vi "Controller - Child 1 -  GET.vi"(8 "error in":errorcluster) -> (0 "error out":errorcluster, 2 "value":dbl)   [LabVIEW 2023, in "Controller.lvlib" / "Controller.lvclass"]
uses:
  Controller.lvclass
  Controller - Ctrl - Actor - Selector.ctl
  GUI/Usr Ev/GUI - Ctrl - Enum - Events.ctl
  GUI/GUI_Class.lvclass
panel:
  in  "Actor Selector":T1=enum."GUI"
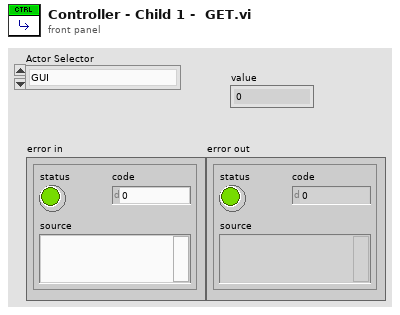
[diagram p1: front panel]
types:
  T1 = typedef "Controller.lvlib/Controller.lvclass/Controller - Ctrl - Actor - Selector.ctl" = enum16{"DISTRIBUTOR", "GUI", "CONSOLE", "SW_INTERFACE", "LOGGING", "ERROR_ENGINE", "EMBEDDED_DB"}
  T2 = typedef "GUI_Actor.lvlib/GUI_Class.lvclass/GUI - Ctrl - Enum - Events.ctl" = enum16{"SEND MESSAGE Ev", "STOP_ACTOR Ev", "INIT_ACTOR Ev", "START Ev", "STOP Ev", "GET Ev", "SET Ev", "ERROR_HANDLER Ev", "RESET Ev", "T2 Ev", "T3 Ev", "T4 Ev"}
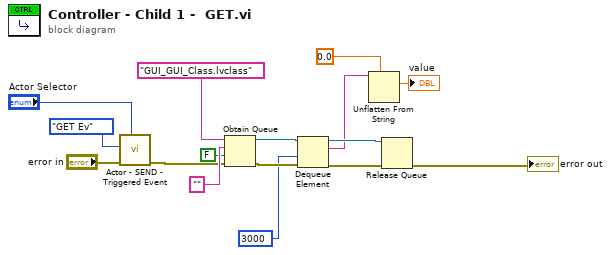
[diagram p0: block diagram]
diagram:
  n1 = call "Actor - SEND - Triggered Event.vi"("Actor Selector"="Actor Selector", "error in (no error)"="error in", "Events"=GUI_-_Ctrl_-_Enum_-_Events."GET Ev") -> ("error out"=w2:errorcluster)  [unwired: 8 in]
  n2 = Obtain Queue(name (unnamed)="GUI_GUI_Class.lvclass", element data type="", create if not found? (T)=FALSE, error in (no error)=w2) -> (queue out=w13:refnum<queue>, error out=w14:errorcluster)  [unwired: 1 in, 1 out]
  n3 = Dequeue Element(queue=w13, timeout in ms (-1)=3000, error in (no error)=w14) -> (queue out=w10:refnum<queue>, element=w9:string, error out=w11:errorcluster)  [unwired: 1 out]
  n4 = Unflatten From String(type=0.0, binary string=w9) -> (value=→"value":dbl)  [unwired: 3 in, 2 out]
  n5 = Release Queue(queue=w10, error in (no error)=w11) -> (error out=→"error out":errorcluster)  [unwired: 1 in, 2 out]
